vi "tcp shot sender wait add connection.vi"(8 "error in (no error)":errorcluster, 10 "timeout ms":i32=100, 11 "Data in":T3) -> (0 "error out":errorcluster, 1 "connected":bool, 2 "connection ID":refnum<k5>, 3 "Data out":T3, 5 "TCPDeviceName":string)   [LabVIEW 2020]
uses:
  tcp shot sender queue.ctl
  TCP Multiple Connections State.ctl
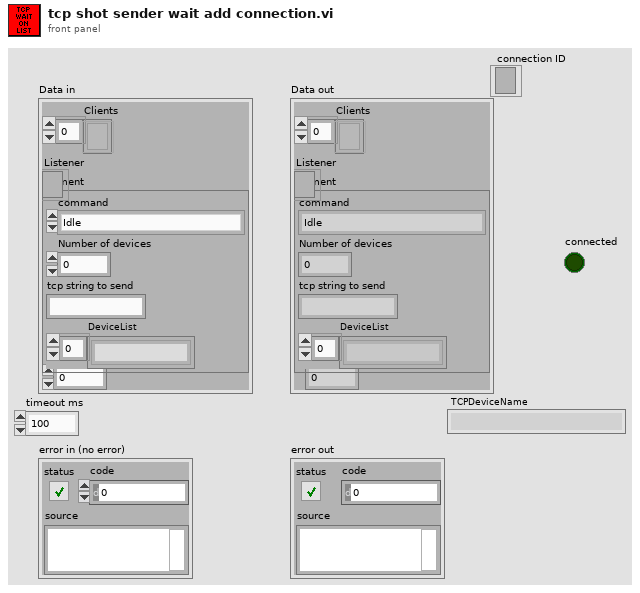
[diagram p1: front panel]
types:
  T1 = typedef "tcp shot sender queue.ctl" = cluster{"command":T2, "Number of devices":i32, "tcp string to send":string, "DeviceList":string[]}
  T2 = typedef "TCP Multiple Connections State.ctl" = enum16{"Idle", "Initialize", "Start Scan", "Send Data", "Stop", "End Scan"}
  T3 = cluster{"Clients":refnum<k5>[], "Listener":refnum<k5>, "element":T1, "startscan tick":u32}
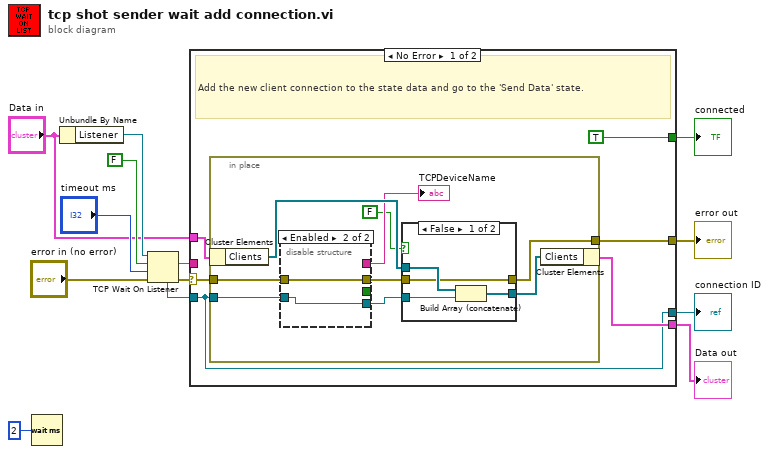
[diagram p0: block diagram]
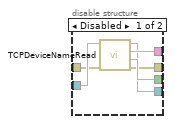
[diagram p2: hidden frame]
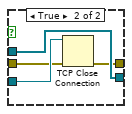
[diagram p3: hidden frame]
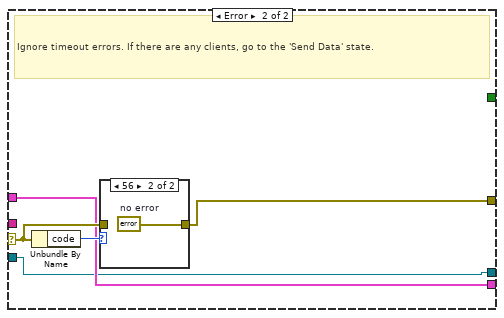
[diagram p4: hidden frame]
diagram:
  n1 = Wait (ms)(milliseconds to wait=u32 2) -> ()  [unwired: 1 out]
  n2 = Unbundle By Name("Data in") -> ("Listener"=w9:refnum<k5>)
  n3 = TCP Wait On Listener(8:"error in (no error)", 9:"timeout ms", 10:FALSE ("resolve remote address (T)"), 11:w9) -> (0:w7:errorcluster, 2:w10:string, 4:w8:refnum<k5>)  [unwired: 2 out]
  n4 = case shown="No Error" w7 {
    selector: w7 -> [w15 w49]
    tunnel: w8 -> [w17 w45]
    tunnel: "Data in" -> [w19 w46]
    tunnel: [w18 w46] -> w13
    tunnel: [w14 w47] -> w11
    tunnel: w10 -> [_ _]
    tunnel: [w17 w45] -> w2
    tunnel: [TRUE ("connected") _] -> w1
    frame No Error {
      # "Add the new client connection to the state data and go to the 'Send Data' state."
      n5 = in-place {
        in-place-border: w17 -> [w26]
        in-place-border: w15 -> [w25]
        in-place-border: [w21] -> w14
        n6 = in-place-cluster #1(w19) -> ("Clients"=w28:refnum<k5>[])
        n7 = disable-structure shown="Enabled" {
          disable-tunnel: w26 -> [w34 w36]
          disable-tunnel: w25 -> [w33 w35]
          disable-tunnel: [w32 _] -> w24
          disable-tunnel: [w31 _] -> _
          disable-tunnel: [w30 w36] -> w23
          disable-tunnel: [w29 w35] -> w22
          frame Disabled {
            n8 = call "TCPDeviceNameRead.vi"("error in (no error)"=w33, "connection ID"=w34) -> ("error out"=w29:errorcluster, "empty?"=w31:bool, "TCPDeviceName"=w32:string, "connection ID out"=w30:refnum<k5>)  [unwired: 6 in]
          }
          frame Enabled {
          }
        }
        "TCPDeviceName" <- w24
        n9 = case shown="False" FALSE {
          tunnel: w28 -> [w40 w44]
          tunnel: [w39 w44] -> w27
          tunnel: w23 -> [w38 w43]
          tunnel: w22 -> [w37 w42]
          tunnel: [w37 w41] -> w21
          frame False {
            n10 = Build Array (concatenate)(w40, w38) -> (w39:refnum<k5>[])
          }
          frame True {
            n11 = TCP Close Connection(connection ID=w43, error in (no error)=w42) -> (error out=w41:errorcluster)  [unwired: 1 in, 1 out]
          }
        }
        n12 = in-place-cluster #1("Clients"=w27) -> (w18:T3)
      }
    }
    frame Error {
      # "Ignore timeout errors. If there are any clients, go to the 'Send Data' state."
      n13 = Unbundle By Name(w49) -> ("code"=w48:i32)
      n14 = case shown="56" w48 {
        tunnel: w49 -> [w50 _]
        tunnel: [w50 w51] -> w47
        frame Default {
        }
        frame 56 {
          w51 = errorcluster {"status"=FALSE, "code"=0, "source"=""}  # no error
        }
      }
    }
  }
  "Data out" <- w13
  "error out" <- w11
  "connection ID" <- w2
  "connected" <- w1
